vi "SP Convert Stimulus Cluster.vi"(4 "Conversion":enum16{"Cluster - HTML", "HTML - Cluster"}(ring), 6 "Stimulus Key Array In":T1, 7 "Stimulus Cluster In":T2={"Use Instrument Settings"=FALSE, "Blank Frequencies"=FALSE, "Sweep Type"=enum."Linear", "Sweep"={"Fstart"=500.0, "Fstop"=1500.0, "Units"=enum."MHz", "Points"=201}, "Power (dBm)"=999.0, "IFBW (Hz)"=-1.0, "Sweep Time (s)"=-1.0, "Calibration"={"State"=FALSE, "String"=""}} {"Sweep Time (s)" format="%.3g"}) -> (1 "Stimulus Cluster Out":T2={"Use Instrument Settings"=FALSE, "Blank Frequencies"=FALSE, "Sweep Type"=enum."Linear", "Sweep"={"Fstart"=0.0, "Fstop"=0.0, "Units"=enum."Hz", "Points"=2}, "Power (dBm)"=999.0, "IFBW (Hz)"=-1.0, "Sweep Time (s)"=-1.0, "Calibration"={"State"=FALSE, "String"=""}} {"Sweep Time (s)" format="%.3g"}, 2 "Stimulus HTML Out":string)   [LabVIEW 2011]
uses:
  TypeDefs/SP Stimulus Parameters.ctl
  TypeDefs/SP Frequency Units.ctl
  TypeDefs/SP Calibration State.ctl
  Addons/internet/utils/keyedarr.llb/Keyed Array.ctl
  Addons/internet/utils/strutil.llb/Case Matching.ctl
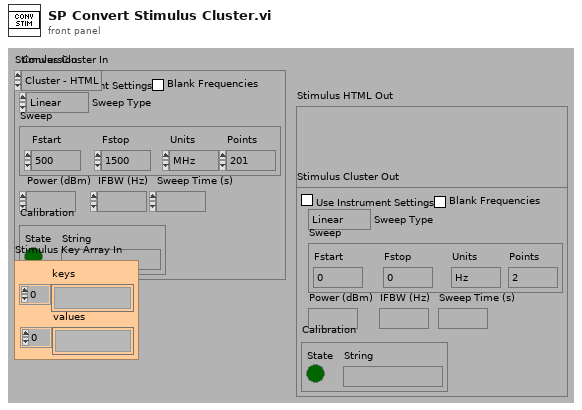
[diagram p1: front panel]
types:
  T1 = typedef "Keyed Array.ctl" = cluster{"keys":string[], "values":string[]}
  T2 = typedef "SP Stimulus Parameters.ctl" = cluster{"Use Instrument Settings":bool, "Blank Frequencies":bool, "Sweep Type":enum32{"Linear", "Logarithmic", "List", "Power", "CW"}, "Sweep":cluster{"Fstart":dbl, "Fstop":dbl, "Units":T3, "Points":i32}, "Power (dBm)":dbl, "IFBW (Hz)":dbl, "Sweep Time (s)":dbl, "Calibration":T4}
  T3 = typedef "SP Frequency Units.ctl" = enum16{"Hz", "kHz", "MHz", "GHz", "Points"}
  T4 = typedef "SP Calibration State.ctl" = cluster{"State":bool, "String":string}
  T5 = enum32{"Linear", "Logarithmic", "List", "Power", "CW"}
  T6 = typedef "Case Matching.ctl" = enum16{"a != A", "a == A", "system"}
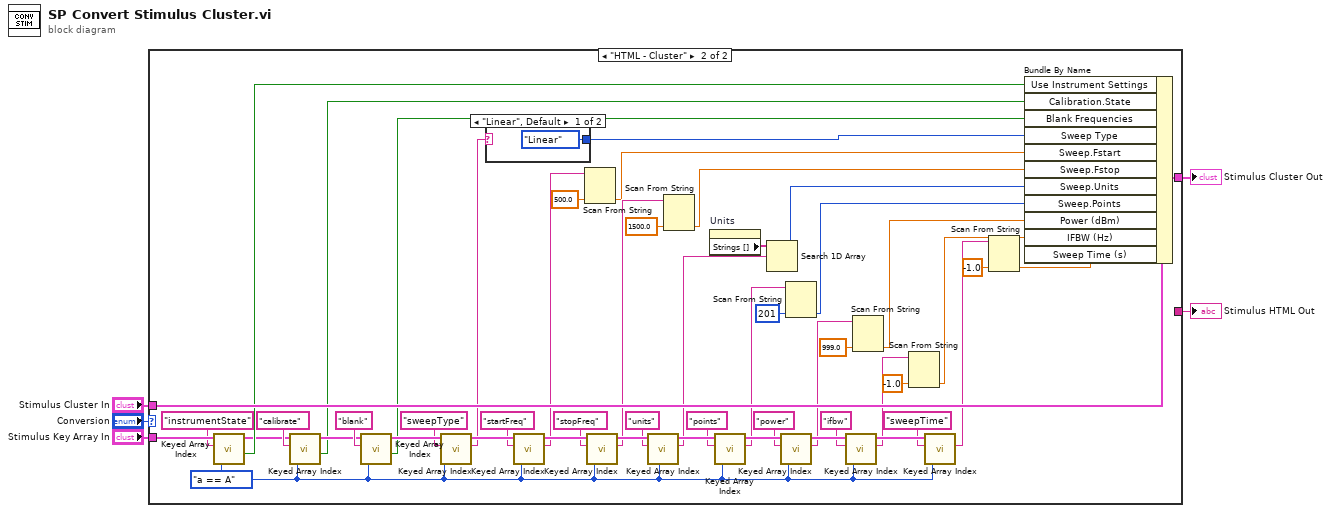
[diagram p0: block diagram]
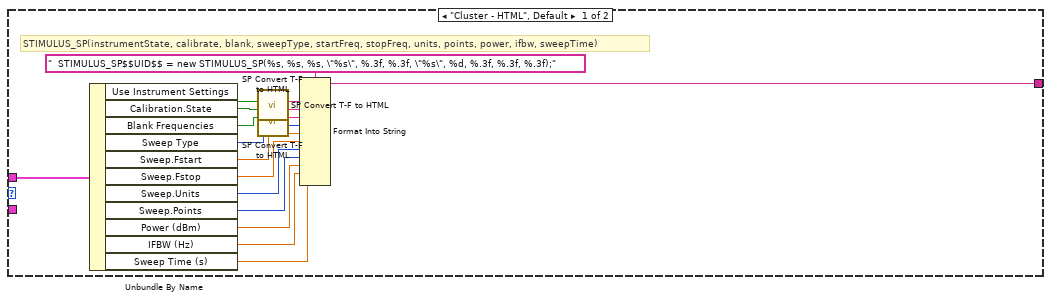
[diagram p2: hidden frame]
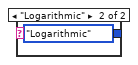
[diagram p3: hidden frame]
diagram:
  n1 = case shown="\"HTML - Cluster\"" "Conversion" {
    tunnel: "Stimulus Cluster In" -> [w22 w54]
    tunnel: "Stimulus Key Array In" -> [_ w73]
    tunnel: [w16 _] -> w2
    tunnel: [_ w35] -> w1
    frame "Cluster - HTML", Default {
      # "STIMULUS_SP(instrumentState, calibrate, blank, sweepType, startFreq, stopFreq, units, points, power, ifbw, sweepTime)"
      n2 = Unbundle By Name(w22) -> ("Use Instrument Settings"=w14:bool, "Calibration.State"=w6:bool, "Blank Frequencies"=w12:bool, "Sweep Type"=w21:T5, "Sweep.Fstart"=w9:dbl, "Sweep.Fstop"=w8:dbl, "Sweep.Units"=w10:T3, "Sweep.Points"=w20:i32, "Power (dBm)"=w19:dbl, "IFBW (Hz)"=w18:dbl, "Sweep Time (s)"=w17:dbl)
      n3 = call "SP Convert T-F to HTML.vi"("(T/F)"=w14) -> ("HTML (true/false)"=w13:string)  [unwired: 10 out]
      n4 = call "SP Convert T-F to HTML.vi"("(T/F)"=w6) -> ("HTML (true/false)"=w7:string)  [unwired: 10 out]
      n5 = call "SP Convert T-F to HTML.vi"("(T/F)"=w12) -> ("HTML (true/false)"=w11:string)  [unwired: 10 out]
      n6 = Format Into String(format string="  STIMULUS_SP$$UID$$ = new STIMULUS_SP(%s, %s, %s, \"%s\", %.3f, %.3f, \"%s\", %d, %.3f, %.3f, %.3f);", w13, w7, w11, w21, w9, w8, w10, w20, w19, w18, w17) -> (resulting string=w16:string)  [unwired: 2 in, 1 out]
    }
    frame "HTML - Cluster" {
      w24 = Case_Matching."a == A" ("case matching (sensitive)")
      n7 = call "Keyed Array Index.vi"("case matching (sensitive)"=w24, "key"="instrumentState", "array in"=w73) -> ("valid key"=w28:bool, "duplicate array"=w26:T1)  [unwired: 1 in, 2 out]
      n8 = call "Keyed Array Index.vi"("case matching (sensitive)"=w24, "key"="calibrate", "array in"=w26) -> ("valid key"=w23:bool, "duplicate array"=w25:T1)  [unwired: 1 in, 2 out]
      n9 = call "Keyed Array Index.vi"("case matching (sensitive)"=w24, "key"="blank", "array in"=w25) -> ("valid key"=w53:bool, "duplicate array"=w71:T1)  [unwired: 1 in, 2 out]
      n10 = call "Keyed Array Index.vi"("case matching (sensitive)"=w24, "key"="sweepType", "array in"=w71) -> ("value"=w52:string, "duplicate array"=w70:T1)  [unwired: 1 in, 2 out]
      n11 = case shown="\"Linear\", Default" w52 {
        tunnel: [T5."Linear" ("Sweep Type") T5."Logarithmic" ("Sweep Type")] -> w29
        frame "Linear", Default {
        }
        frame "Logarithmic" {
        }
      }
      n12 = call "Keyed Array Index.vi"("case matching (sensitive)"=w24, "key"="startFreq", "array in"=w70) -> ("value"=w51:string, "duplicate array"=w69:T1)  [unwired: 1 in, 2 out]
      n13 = Scan From String(input string=w51, default 1=500.0 ("default value 1")) -> (output 1=w31:dbl)  [unwired: 3 in, 3 out]
      n14 = call "Keyed Array Index.vi"("case matching (sensitive)"=w24, "key"="stopFreq", "array in"=w69) -> ("value"=w48:string, "duplicate array"=w68:T1)  [unwired: 1 in, 2 out]
      n15 = call "Keyed Array Index.vi"("case matching (sensitive)"=w24, "key"="units", "array in"=w68) -> ("value"=w32:string, "duplicate array"=w67:T1)  [unwired: 1 in, 2 out]
      n16 = Scan From String(input string=w48, default 1=1500.0 ("default value 1")) -> (output 1=w30:dbl)  [unwired: 3 in, 3 out]
      n17 = property on="Units" class="Enum (strict)"() -> ("Strings []"=w33:string[])  [unwired: 2 in, 2 out]
      n18 = call "Keyed Array Index.vi"("case matching (sensitive)"=w24, "key"="points", "array in"=w67) -> ("value"=w46:string, "duplicate array"=w66:T1)  [unwired: 1 in, 2 out]
      n19 = Search 1D Array(1D array=w33, element=w32) -> (index of element=w34:i32)  [unwired: 1 out]
      n20 = call "Keyed Array Index.vi"("case matching (sensitive)"=w24, "key"="power", "array in"=w66) -> ("value"=w43:string, "duplicate array"=w65:T1)  [unwired: 1 in, 2 out]
      n21 = Scan From String(input string=w46, default 1=201 ("default value 1")) -> (output 1=w45:i32)  [unwired: 3 in, 3 out]
      n22 = call "Keyed Array Index.vi"("case matching (sensitive)"=w24, "key"="ifbw", "array in"=w65) -> ("value"=w39:string, "duplicate array"=w64:T1)  [unwired: 1 in, 2 out]
      n23 = Scan From String(input string=w43, default 1=999.0 ("default value 1")) -> (output 1=w42:dbl)  [unwired: 3 in, 3 out]
      n24 = Scan From String(input string=w39, default 1=-1.0 ("default value 1")) -> (output 1=w38:dbl)  [unwired: 3 in, 3 out]
      n25 = call "Keyed Array Index.vi"("case matching (sensitive)"=w24, "key"="sweepTime", "array in"=w64) -> ("value"=w37:string)  [unwired: 1 in, 3 out]
      n26 = Scan From String(input string=w37, default 1=-1.0 ("default value 1")) -> (output 1=w36:dbl)  [unwired: 3 in, 3 out]
      n27 = Bundle By Name(cluster=w54, "Use Instrument Settings"=w28, "Calibration.State"=w23, "Blank Frequencies"=w53, "Sweep Type"=w29, "Sweep.Fstart"=w31, "Sweep.Fstop"=w30, "Sweep.Units"=w34, "Sweep.Points"=w45, "Power (dBm)"=w42, "IFBW (Hz)"=w38, "Sweep Time (s)"=w36) -> (w35:T2)
    }
  }
  "Stimulus HTML Out" <- w2
  "Stimulus Cluster Out" <- w1
